vi "Filter non-ascii characters.vi"(1 "bypass":bool, 2 "?":string) -> (0 "output":string)   [LabVIEW 2021]
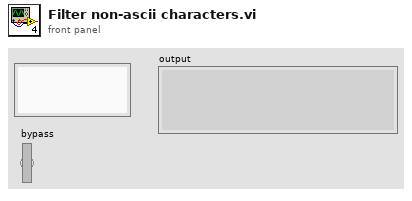
[diagram p1: front panel]
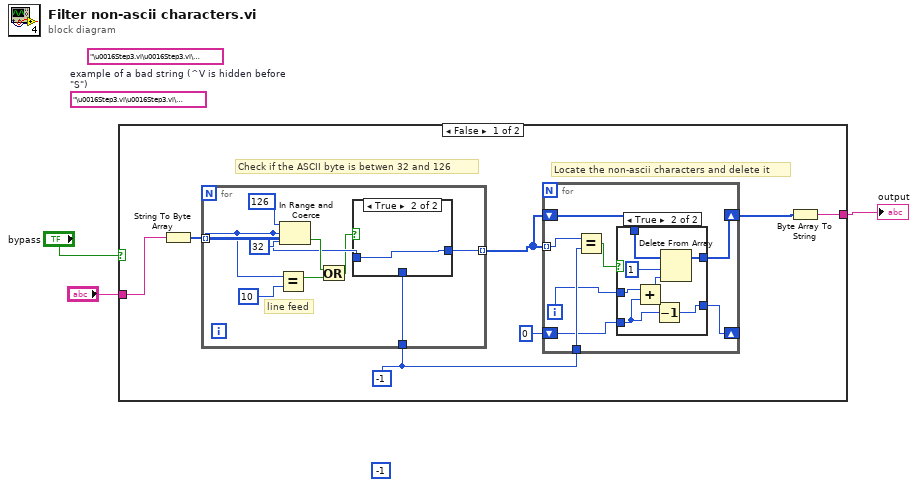
[diagram p0: block diagram]
diagram:
  (unwired) i8 -1
  (unwired) "\u0016Step3.vi\u0016Step3.vi\u0016Step3.vi"  # example of a bad string (^V is hidden before "S")
  (unwired) "\u0016Step3.vi\u0016Step3.vi\u0016Step3.vi"
  n1 = case shown="False" "bypass" {
    tunnel: [w9 w39] -> w3
    tunnel: "?" -> [w4 w39]
    frame False {
      w8 = i8 -1
      # "Locate the non-ascii characters and delete it"
      # "Check if the ASCII byte is betwen 32 and 126"
      n2 = String To Byte Array(string=w4) -> (unsigned byte array=w10:u8[])
      n3 = for {
        tunnel: w10 -> [w31] mode=indexing
        tunnel: [w35] -> w7 mode=indexing
        tunnel: w8 -> [w36]
        # "line feed"
        n4 = Equal?(x=w31, y=u8 10) -> (x = y?=w29:bool)
        n5 = In Range and Coerce(upper limit=u8 126, x=w31, lower limit=u8 32) -> (In Range?=w32:bool)  [unwired: 1 out]
        n6 = Or(x=w32, y=w29) -> (x .or. y?=w28:bool)
        n7 = case shown="True" w28 {
          tunnel: [w37 w38] -> w35
          tunnel: w36 -> [w37 _]
          tunnel: w31 -> [_ w38]
          frame False {
          }
          frame True {
          }
        }
      }
      n8 = for {
        tunnel: w7 -> [w18] mode=indexing
        tunnel: w8 -> [w17]
        shift-right: [w14] -> w6
        shift-left: w7 -> [w16]
        shift-right: [w11] -> _
        shift-left: i8 0 -> [w13]
        i -> [w15]
        n9 = Equal?(x=w18, y=w17) -> (x = y?=w12:bool)
        n10 = case shown="True" w12 {
          tunnel: w16 -> [w20 w27]
          tunnel: w15 -> [_ w23]
          tunnel: [w20 w25] -> w14
          tunnel: w13 -> [w19 w21]
          tunnel: [w19 w24] -> w11
          frame False {
          }
          frame True {
            n11 = Add(x=w23, y=w21) -> (x+y=w22:i32)
            n12 = Decrement(x=w21) -> (x-1=w24:i8)
            n13 = Delete From Array(array=w27, length=1, index=w22) -> (array with subset deleted=w25:u8[])  [unwired: 1 out]
          }
        }
      }
      n14 = Byte Array To String(unsigned byte array=w6) -> (string=w9:string)
    }
    frame True {
    }
  }
  "output" <- w3
